vi "I2C Read Write Relay Control.vi"(8 "error in (no error)":errorcluster, 10 "deviceAddress":u8=32 format="%x", 11 "handle":u64 format="%x") -> (0 "error out":errorcluster, 2 "sizeTransferred":u32, 3 "handle 2":u64 format="%x")   [LabVIEW 2024, in "libMPSSE-I2C.lvlib"]
uses:
  libMPSSE-I2C.lvlib
  libmpsse.dll
panel:
  out "return (Low)":u64
  out "return (Output)":u64
  out "return type":u64
  out "sizeTransferred (Low)":u32
  out "return (High)":u64
  out "sizeTransferred (High)":u32
  out "sizeTransferred (Output)":u32
  # "Write = Set as Ouput\n          = Set as High\n          = Set as Low"
  # "Input"
  # "Read Results"
  # "* ALL Data is inputted as hex decimal"
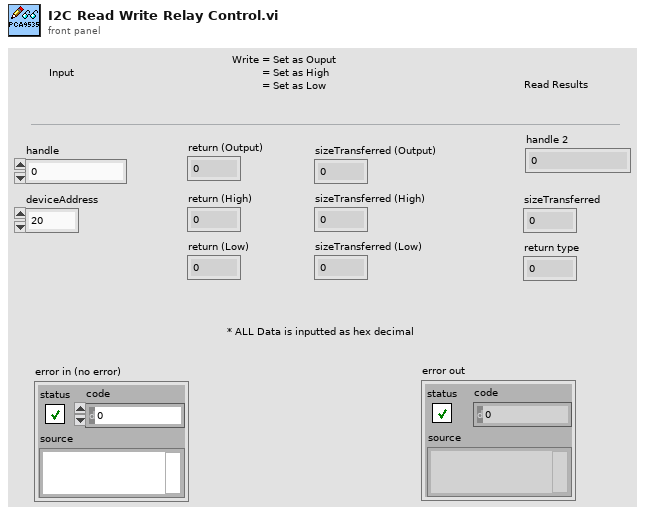
[diagram p1: front panel]
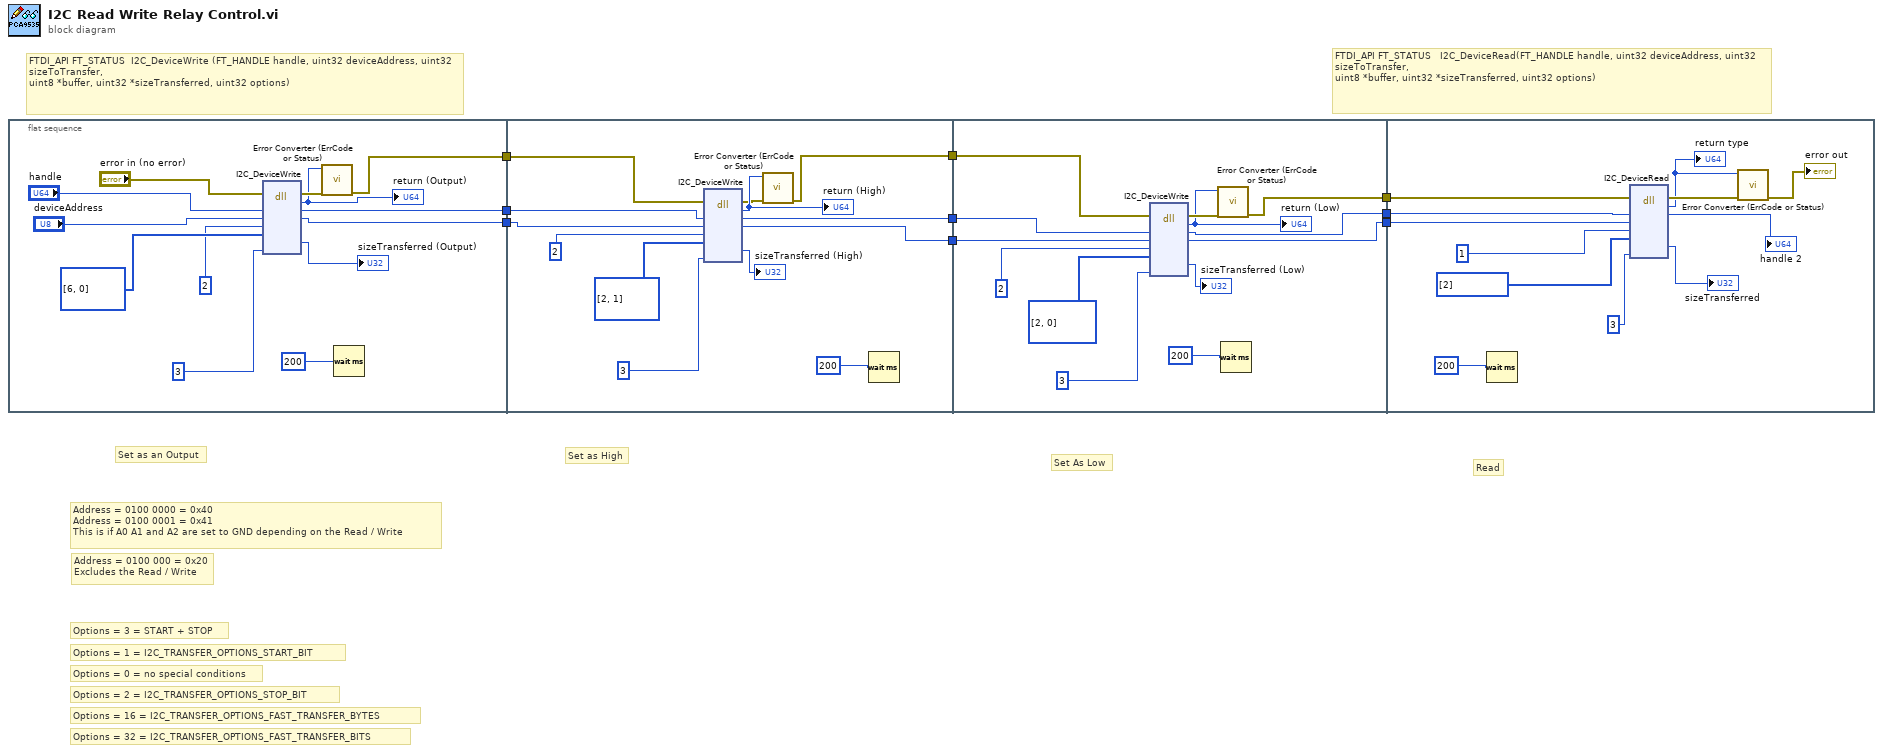
[diagram p0: block diagram]
diagram:
  # "Address = 0100 000 = 0x20\nExcludes the Read / Write"
  # "Options = 3 = START + STOP"
  # "Address = 0100 0000 = 0x40\nAddress = 0100 0001 = 0x41\nThis is if A0 A1 and A2 are set to GND depending on the Read / Write"
  # "Options = 32 = I2C_TRANSFER_OPTIONS_FAST_TRANSFER_BITS"
  # "Options = 16 = I2C_TRANSFER_OPTIONS_FAST_TRANSFER_BYTES"
  # "Options = 2 = I2C_TRANSFER_OPTIONS_STOP_BIT"
  # "Options = 0 = no special conditions"
  # "Options = 1 = I2C_TRANSFER_OPTIONS_START_BIT"
  # "Read"
  # "Set As Low"
  # "Set as High"
  # "Set as an Output"
  # "FTDI_API FT_STATUS   I2C_DeviceRead(FT_HANDLE handle, uint32 deviceAddress, uint32 sizeToTransfer, \nuint8 *buffer, uint32 *sizeTransferred, uint32 options)"
  # "FTDI_API FT_STATUS  I2C_DeviceWrite (FT_HANDLE handle, uint32 deviceAddress, uint32 sizeToTransfer, \nuint8 *buffer, uint32 *sizeTransferred, uint32 options)"
  n1 = flat-sequence {
    tunnel: [w20] -> w9
    tunnel: [w19] -> w8
    tunnel: [w16] -> w3
    tunnel: w9 -> [w24]
    tunnel: w8 -> [w23]
    tunnel: [w30] -> w6
    tunnel: [w29] -> w4
    tunnel: w3 -> [w27]
    tunnel: [w26] -> w2
    tunnel: [w44] -> w7
    tunnel: w6 -> [w43]
    tunnel: [w42] -> w5
    tunnel: w4 -> [w41]
    tunnel: w2 -> [w39]
    tunnel: [w38] -> w1
    tunnel: w7 -> [w56]
    tunnel: w5 -> [w55]
    tunnel: w1 -> [w52]
    frame #0 {
      n2 = dll-call lib="C:/Workspace/sm_6576_001_RIB_Sequencer/I2C/libmpsse.dll" fn="I2C_DeviceWrite"(error in="error in (no error)", "handle"="handle", "deviceAddress"="deviceAddress", "sizeToTransfer"=u16 2, "buffer"=u8[] [6, 0] ("*buffer 4"), "options"=u32 3) -> (error out=w21:errorcluster, "return type"=w13:u64, "handle"=w20:u64, "deviceAddress"=w19:u8, "sizeTransferred"=→"sizeTransferred (Output)":u32)  [unwired: 6 in, 1 out]
      "return (Output)" <- w13
      n3 = call "Error Converter (ErrCode or Status).vi"("error in (no error)"=w21, "error code"=w13) -> ("error out"=w16:errorcluster)  [unwired: 9 in]
      n4 = Wait (ms)(milliseconds to wait=u32 200) -> ()  [unwired: 1 out]
    }
    frame #1 {
      n5 = dll-call lib="C:/Workspace/sm_6576_001_RIB_Sequencer/I2C/libmpsse.dll" fn="I2C_DeviceWrite"(error in=w27, "handle"=w24, "deviceAddress"=w23, "sizeToTransfer"=u32 2, "buffer"=u8[] [2, 1] ("*buffer 4"), "options"=u32 3) -> (error out=w34:errorcluster, "return type"=w35:u64, "handle"=w30:u64, "deviceAddress"=w29:u8, "sizeTransferred"=→"sizeTransferred (High)":u32)  [unwired: 6 in, 1 out]
      "return (High)" <- w35
      n6 = call "Error Converter (ErrCode or Status).vi"("error in (no error)"=w34, "error code"=w35) -> ("error out"=w26:errorcluster)  [unwired: 9 in]
      n7 = Wait (ms)(milliseconds to wait=u32 200) -> ()  [unwired: 1 out]
    }
    frame #2 {
      n8 = dll-call lib="C:/Workspace/sm_6576_001_RIB_Sequencer/I2C/libmpsse.dll" fn="I2C_DeviceWrite"(error in=w39, "handle"=w43, "deviceAddress"=w41, "sizeToTransfer"=u32 2, "buffer"=u8[] [2, 0] ("*buffer 5"), "options"=u32 3) -> (error out=w48:errorcluster, "return type"=w36:u64, "handle"=w44:u64, "deviceAddress"=w42:u8, "sizeTransferred"=→"sizeTransferred (Low)":u32)  [unwired: 6 in, 1 out]
      "return (Low)" <- w36
      n9 = call "Error Converter (ErrCode or Status).vi"("error in (no error)"=w48, "error code"=w36) -> ("error out"=w38:errorcluster)  [unwired: 9 in]
      n10 = Wait (ms)(milliseconds to wait=u32 200) -> ()  [unwired: 1 out]
    }
    frame #3 {
      n11 = Wait (ms)(milliseconds to wait=u32 200) -> ()  [unwired: 1 out]
      n12 = dll-call lib="C:/Workspace/sm_6576_001_RIB_Sequencer/I2C/libmpsse.dll" fn="I2C_DeviceRead"(error in=w52, "handle"=w56, "deviceAddress"=w55, "sizeToTransfer"=u32 1 ("sizeToTransfer 3"), "buffer"=u8[] [2] ("*buffer 3"), "options"=u32 3) -> (error out=w57:errorcluster, "return type"=w50:u64, "handle"=→"handle 2":u64, "sizeTransferred"=→"sizeTransferred":u32)  [unwired: 7 in, 1 out]
      "return type" <- w50
      n13 = call "Error Converter (ErrCode or Status).vi"("error in (no error)"=w57, "error code"=w50) -> ("error out"=→"error out":errorcluster)  [unwired: 9 in]
    }
  }
